vi "EnvMillikOpen.vi"(8 "error in (no error)":errorcluster, 10 "Read Timeout":u32=1000, 11 "VISA resource name":refnum<visa-resource-name>="COM3") -> (0 "error out":errorcluster, 3 "VISA resource name out":refnum<visa-resource-name>)   [LabVIEW 2016]
uses:
  <vilib>/Instr/_visa.llb/VISA Flush IO Buffer Mask.ctl
  <vilib>/Instr/_visa.llb/Select Event Type.ctl
panel:
  out "return count 3":u32
  out "concatenated string 2":string
  out "return count 2":u32
  out "substring 2":string
  out "read buffer 2":string
  out "concatenated string":string
  out "return count":u32
  out "read buffer":string
  out "substring":string
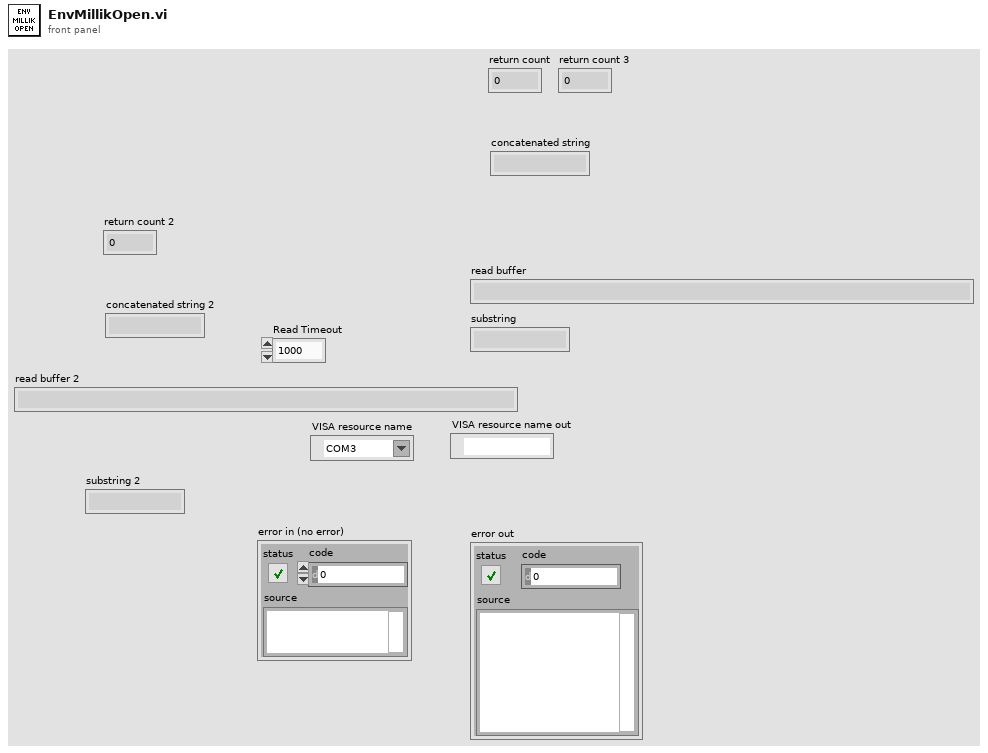
[diagram p1: front panel]
types:
  T1 = typedef "VISA Flush IO Buffer Mask.ctl" = u16
  T2 = typedef "Select Event Type.ctl" = u32
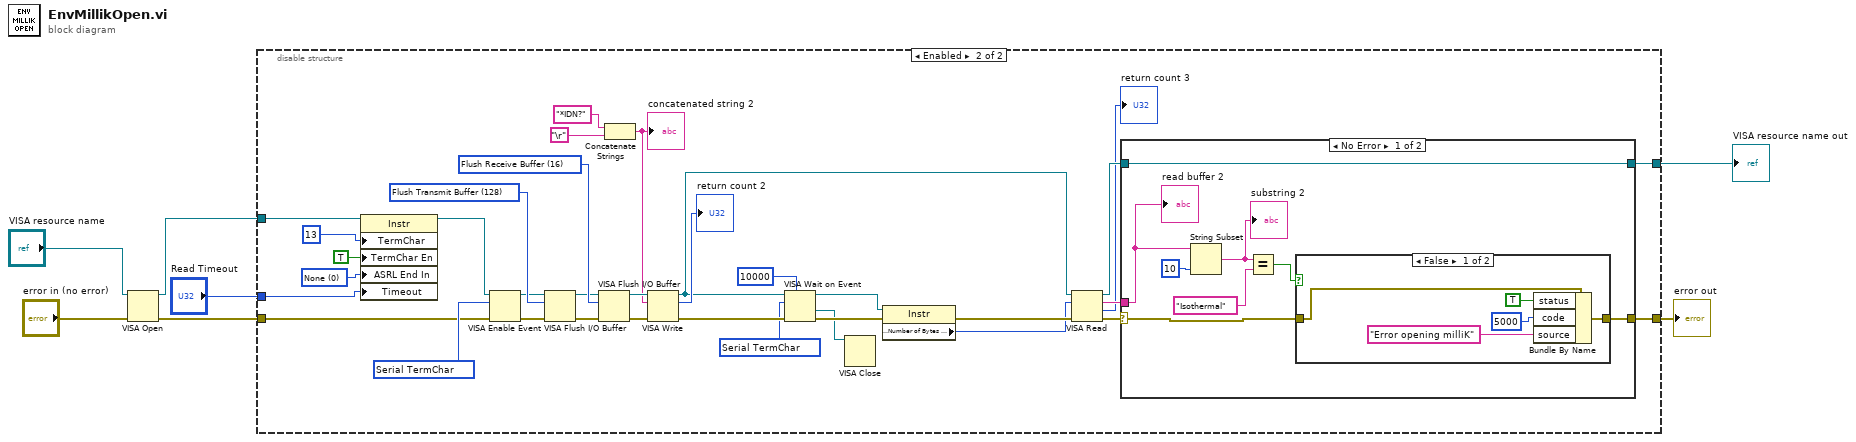
[diagram p0: block diagram]
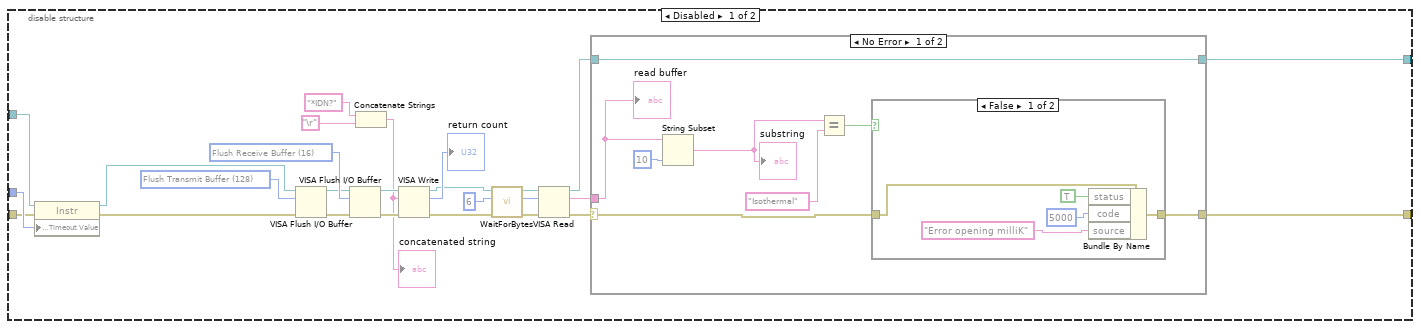
[diagram p2: hidden frame]
diagram:
  n1 = VISA Open(error in (no error)="error in (no error)", VISA resource name="VISA resource name") -> (VISA resource name=w5:refnum<visa-resource-name>, error out=w4:errorcluster)  [unwired: 3 in]
  n2 = disable-structure shown="Enabled" {
    disable-tunnel: "Read Timeout" -> [w33 w55]
    disable-tunnel: w5 -> [w32 w62]
    disable-tunnel: w4 -> [w31 w58]
    disable-tunnel: [w30 w70] -> w2
    disable-tunnel: [w29 w71] -> w3
    frame Disabled {
      w26 = T1 128 items=["Flush Receive Buffer"=16, "Write Transmit Buffer to Device"=32, "Flush Receive Buffer (No I/O)"=64, "Flush Transmit Buffer"=128] ("Mask")
      w27 = T1 16 items=["Flush Receive Buffer"=16, "Write Transmit Buffer to Device"=32, "Flush Receive Buffer (No I/O)"=64, "Flush Transmit Buffer"=128] ("Mask")
      n3 = property class="Instr"(reference=w32, error in=w31, "General Settings:Timeout Value"=w33) -> (reference out=w22:refnum<visa-resource-name>, error out=w23:errorcluster)
      n4 = VISA Flush I/O Buffer(VISA resource name=w22, mask (16)=w26, error in (no error)=w23) -> (VISA resource name out=w25:refnum<visa-resource-name>, error out=w24:errorcluster)
      n5 = VISA Flush I/O Buffer(VISA resource name=w25, mask (16)=w27, error in (no error)=w24) -> (VISA resource name out=w21:refnum<visa-resource-name>, error out=w20:errorcluster)
      n6 = Concatenate Strings("*IDN?" ("write buffer"), "\r") -> (w17:string)
      "concatenated string" <- w17
      n7 = VISA Write(VISA resource name=w21, write buffer=w17, error in (no error)=w20) -> (VISA resource name out=w14:refnum<visa-resource-name>, return count=→"return count":u32, error out=w13:errorcluster)
      n8 = call "WaitForBytes.vi"("error in (no error)"=w13, "timeout [s]"=6, "VISA Refnum in"=w14) -> ("error out"=w16:errorcluster, "Bytes at Port"=w11:u32, "VISA Refnum out"=w15:refnum<visa-resource-name>)  [unwired: 6 in]
      n9 = VISA Read(VISA resource name=w15, byte count=w11, error in (no error)=w16) -> (VISA resource name out=w10:refnum<visa-resource-name>, read buffer=w9:string, error out=w8:errorcluster)  [unwired: 1 out]
      n10 = case shown="No Error" w8 {
        selector: w8 -> [w36 w49]
        tunnel: [w37 w49] -> w29
        tunnel: w10 -> [w35 w48]
        tunnel: [w35 w48] -> w30
        tunnel: w9 -> [w34 _]
        frame No Error {
          n11 = String Subset(string=w34, length (rest)=10 ("length (rest)")) -> (substring=w40:string)  [unwired: 1 in]
          "substring" <- w40
          n12 = Equal?(x=w40, y="Isothermal" ("true string")) -> (x = y?=w38:bool)
          n13 = case shown="False" w38 {
            tunnel: w36 -> [w46 w47]
            tunnel: [w43 w47] -> w37
            frame False {
              n14 = Bundle By Name(cluster=w46, "status"=TRUE, "code"=5000, "source"="Error opening milliK") -> (w43:errorcluster)
            }
            frame True {
            }
          }
          "read buffer" <- w34
        }
        frame Error {
        }
      }
    }
    frame Enabled {
      w50 = T2 1073684516 items=["Service Request"=1073684491, "Trigger"=3221168138, "Clear"=1073684493, "VXI Signal"=1073684512, "VXI/VME Interrupt"=3221168161, "VXI/VME Sysfail"=1073684509, "VXI/VME Sysreset"=1073684510, "GPIB CIC"=1073684498, "GPIB Talk"=1073684499, "GPIB Listen"=1073684500, "PXI Interrupt"=1073684514, "Serial Break"=1073684515, "Serial TermChar"=1073684516, "Serial CTS"=1073684521, "Serial DSR"=1073684522, "Serial DCD"=1073684524, "Serial RI"=1073684526, "Serial Character"=1073684533, "USB Interrupt"=1073684535, "All Enabled"=1073709055] ("Event Type")
      w61 = T2 1073684516 items=["Service Request"=1073684491, "Trigger"=3221168138, "Clear"=1073684493, "VXI Signal"=1073684512, "VXI/VME Interrupt"=3221168161, "VXI/VME Sysfail"=1073684509, "VXI/VME Sysreset"=1073684510, "GPIB CIC"=1073684498, "GPIB Talk"=1073684499, "GPIB Listen"=1073684500, "PXI Interrupt"=1073684514, "Serial Break"=1073684515, "Serial TermChar"=1073684516, "Serial CTS"=1073684521, "Serial DSR"=1073684522, "Serial DCD"=1073684524, "Serial RI"=1073684526, "Serial Character"=1073684533, "USB Interrupt"=1073684535, "All Enabled"=1073709055] ("Event Type")
      w63 = u16 0 items=["None", "Last Bit", "TermChar"] ("Serial Settings:End Mode for Reads")
      w82 = T1 128 items=["Flush Receive Buffer"=16, "Write Transmit Buffer to Device"=32, "Flush Receive Buffer (No I/O)"=64, "Flush Transmit Buffer"=128] ("Mask")
      w83 = T1 16 items=["Flush Receive Buffer"=16, "Write Transmit Buffer to Device"=32, "Flush Receive Buffer (No I/O)"=64, "Flush Transmit Buffer"=128] ("Mask")
      n15 = property class="Instr"(reference=w62, "TermChar"=u8 13 ("Message Based Settings:Termination Character"), "TermChar En"=TRUE ("Message Based Settings:Termination Character Enable"), "ASRL End In"=w63, "Timeout"=w55) -> (reference out=w60:refnum<visa-resource-name>)  [unwired: 1 in, 1 out]
      n16 = VISA Enable Event(8:w58, 10:w61, 11:w60) -> (0:w57:errorcluster, 3:w59:refnum<visa-resource-name>)  [unwired: 1 in]
      n17 = VISA Flush I/O Buffer(VISA resource name=w59, mask (16)=w82, error in (no error)=w57) -> (VISA resource name out=w81:refnum<visa-resource-name>, error out=w80:errorcluster)
      n18 = VISA Flush I/O Buffer(VISA resource name=w81, mask (16)=w83, error in (no error)=w80) -> (VISA resource name out=w79:refnum<visa-resource-name>, error out=w78:errorcluster)
      n19 = Concatenate Strings("*IDN?" ("write buffer"), "\r") -> (w75:string)
      "concatenated string 2" <- w75
      n20 = VISA Write(VISA resource name=w79, write buffer=w75, error in (no error)=w78) -> (VISA resource name out=w65:refnum<visa-resource-name>, return count=→"return count 2":u32, error out=w69:errorcluster)
      n21 = VISA Wait on Event(7:u32 10000 ("timeout (0)"), 8:w69, 10:w50, 11:w65) -> (0:w53:errorcluster, 1:w52:refnum<visa-resource-name>, 3:w54:refnum<visa-resource-name>)  [unwired: 1 in, 1 out]
      n22 = VISA Close(VISA resource name=w52) -> ()  [unwired: 1 in, 1 out]
      n23 = property class="Instr"(reference=w54, error in=w53) -> (error out=w68:errorcluster, "Serial Settings:Number of Bytes at Serial Port"=w56:u32)  [unwired: 1 out]
      n24 = VISA Read(VISA resource name=w65, byte count=w56, error in (no error)=w68) -> (VISA resource name out=w74:refnum<visa-resource-name>, read buffer=w73:string, return count=→"return count 3":u32, error out=w72:errorcluster)
      n25 = case shown="No Error" w72 {
        selector: w72 -> [w87 w100]
        tunnel: [w88 w100] -> w71
        tunnel: w74 -> [w86 w99]
        tunnel: [w86 w99] -> w70
        tunnel: w73 -> [w85 _]
        frame No Error {
          n26 = String Subset(string=w85, length (rest)=10 ("length (rest)")) -> (substring=w91:string)  [unwired: 1 in]
          "substring 2" <- w91
          n27 = Equal?(x=w91, y="Isothermal" ("true string")) -> (x = y?=w89:bool)
          n28 = case shown="False" w89 {
            tunnel: w87 -> [w97 w98]
            tunnel: [w94 w98] -> w88
            frame False {
              n29 = Bundle By Name(cluster=w97, "status"=TRUE, "code"=5000, "source"="Error opening milliK") -> (w94:errorcluster)
            }
            frame True {
            }
          }
          "read buffer 2" <- w85
        }
        frame Error {
        }
      }
    }
  }
  "error out" <- w3
  "VISA resource name out" <- w2
